vi "prueba.vi"() -> ()   [LabVIEW 2023]
uses:
  <vilib>/Instr/_visa.llb/VISA Configure Serial Port (Instr).vi
panel:
  in  "Tiempo":u32
  in  "stop":bool
  out "read buffer":string
  out "Waveform Chart":dynamicdata(graph)
  out "number":dbl
  out "number 2":dbl
  in  "VISA resource name":refnum<visa-resource-name>
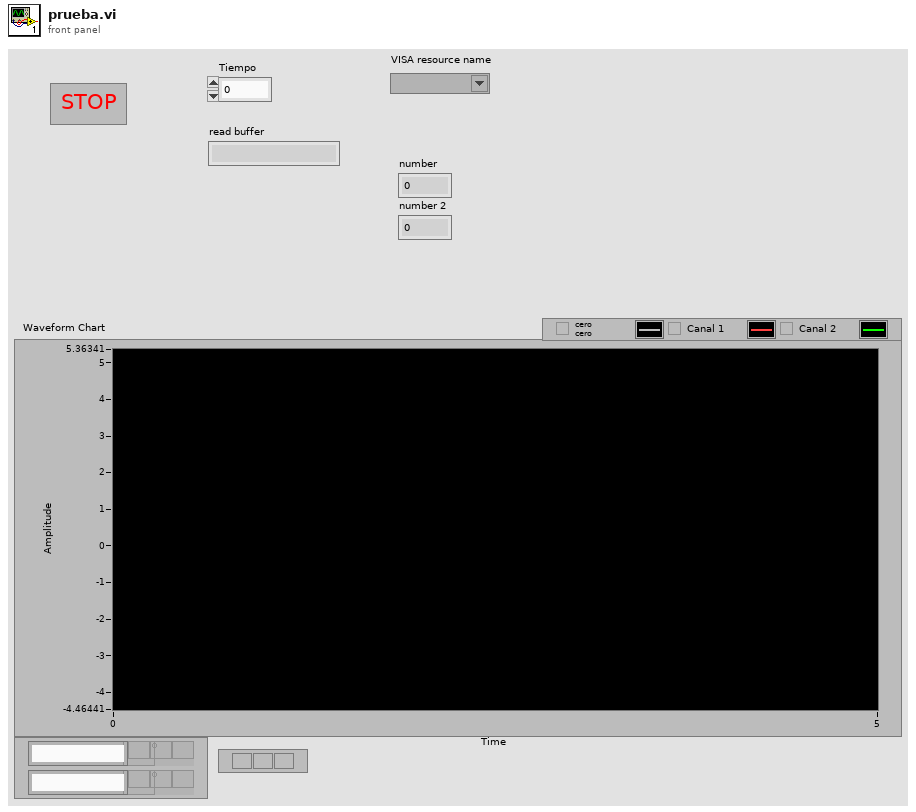
[diagram p1: front panel]
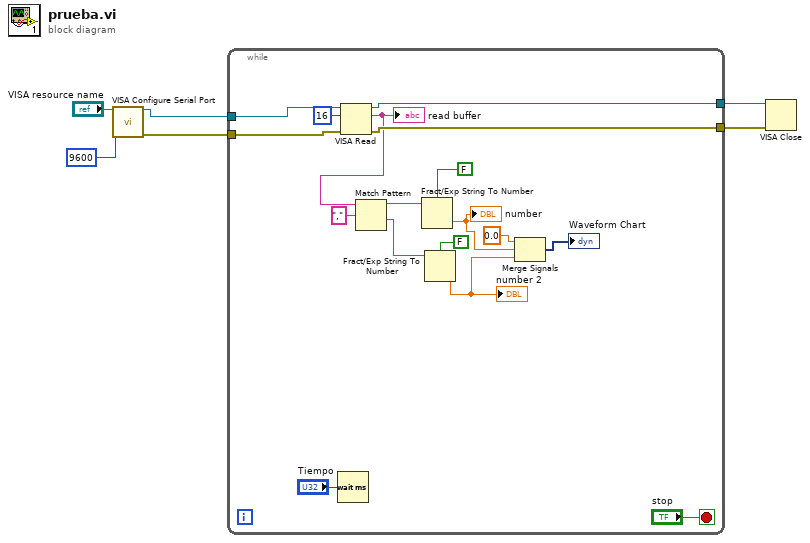
[diagram p0: block diagram]
diagram:
  n1 = call-poly "VISA Configure Serial Port"("VISA resource name"="VISA resource name", "baud rate (9600)"=u32 9600) -> ("VISA resource name out"=w5:refnum<visa-resource-name>, "error out"=w4:errorcluster)  [unwired: 12 in]
  n2 = while {
    tunnel: w5 -> [w23]
    tunnel: w4 -> [w22]
    tunnel: [w21] -> w3
    tunnel: [w20] -> w2
    stop <- "stop" stop-if-true
    n3 = Wait (ms)(milliseconds to wait="Tiempo") -> ()  [unwired: 1 out]
    n4 = VISA Read(VISA resource name=w23, byte count=u32 16, error in (no error)=w22) -> (VISA resource name out=w21:refnum<visa-resource-name>, read buffer=w14:string, error out=w20:errorcluster)  [unwired: 1 out]
    "read buffer" <- w14
    n5 = Match Pattern(string=w14, regular expression=",") -> (before substring=w12:string, after substring=w11:string)  [unwired: 1 in, 2 out]
    n6 = Fract/Exp String To Number(use system decimal point (T)=FALSE, string=w12) -> (number=w8:dbl)  [unwired: 2 in, 1 out]
    "number" <- w8
    n7 = Fract/Exp String To Number(use system decimal point (T)=FALSE, string=w11) -> (number=w9:dbl)  [unwired: 2 in, 1 out]
    "number 2" <- w9
    n8 = Merge Signals(0.0, w8, w9) -> (→"Waveform Chart":dynamicdata)
  }
  n9 = VISA Close(VISA resource name=w3, error in (no error)=w2) -> ()  [unwired: 1 out]
